vi "NewVIObjectOwnerByUID.vi"(4 "bounds":T1, 5 "vi object class":refnum<vi>, 6 "location":T2, 7 "style":i32, 8 "error in (no error)":errorcluster, 10 "owner":cluster{"owner?":bool, "ownerUID":i32}, 11 "targetVI":refnum<vi>) -> (0 "error out":errorcluster, 1 "UID":i32, 2 "object refnum":refnum<vi>, 3 "dup targetVI":refnum<vi>)   [LabVIEW 2013]
uses:
  <vilib>/Utility/miscctls.llb/LVPointTypeDef.ctl
  <vilib>/Utility/miscctls.llb/LVBoundsTypeDef.ctl
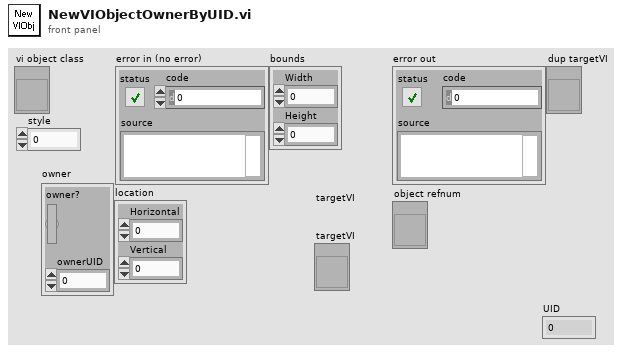
[diagram p1: front panel]
types:
  T1 = typedef "LVBoundsTypeDef.ctl" = cluster{"Width":u32, "Height":u32}
  T2 = typedef "LVPointTypeDef.ctl" = cluster{"Horizontal":i16, "Vertical":i16}
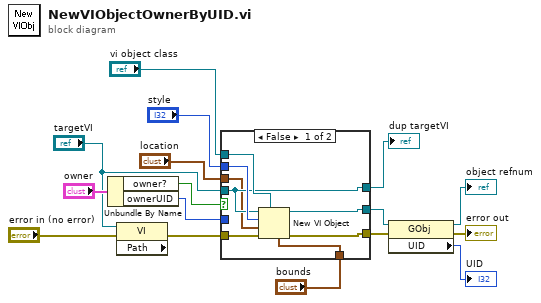
[diagram p0: block diagram]
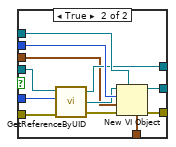
[diagram p2: hidden frame]
diagram:
  n1 = Unbundle By Name("owner") -> ("owner?"=w16:bool, "ownerUID"=w15:i32)
  n2 = property class="VI" props=["Path"](reference="targetVI", error in="error in (no error)") -> (error out=w3:errorcluster)  [unwired: 2 out]
  n3 = case shown="False" w16 {
    tunnel: w3 -> [w23 w35]
    tunnel: "targetVI" -> [w19 w36]
    tunnel: w15 -> [_ w34]
    tunnel: [w24 w27] -> w6
    tunnel: [w21 w32] -> w9
    tunnel: "vi object class" -> [w20 w31]
    tunnel: "style" -> [w22 w30]
    tunnel: [w19 w28] -> w11
    tunnel: "location" -> [w18 w26]
    tunnel: "bounds" -> [w17 w25]
    frame False {
      n4 = New VI Object(vi object class=w20, owner refnum=w19, style=w22, position/next to=w18, 4:w17, 8:w23) -> (object refnum=w21:refnum<vi>, 0:w24:errorcluster)  [unwired: 2 in]
    }
    frame True {
      n5 = call "GetReferenceByUID.vi"("error in (no error)"=w35, "UID"=w34, "targetVI"=w36) -> ("error out"=w33:errorcluster, "refNum"=w29:refnum<vi>, "dup targetVI"=w28:refnum<vi>)  [unwired: 1 in]
      n6 = New VI Object(vi object class=w31, owner refnum=w29, style=w30, position/next to=w26, 4:w25, 8:w33) -> (object refnum=w32:refnum<vi>, 0:w27:errorcluster)  [unwired: 2 in]
    }
  }
  "dup targetVI" <- w11
  n7 = property class="GObj"(reference=w9, error in=w6) -> (reference out=→"object refnum":refnum<vi>, error out=→"error out":errorcluster, "UID"=→"UID":i32)
